vi "Configure Time Interval Gate.vi"(8 "error in (no error)":errorcluster, 9 "Gate Polarity (1: Negative)":i32(ring)=1 items=["Positive", "Negative"], 10 "Gate Source (0: Immediate)":i32(ring) items=["Immediate", "External", "Advanced"], 11 "VISA resource name":refnum<visa-resource-name>) -> (0 "error out":errorcluster, 3 "VISA resource name out":refnum<visa-resource-name>)   [LabVIEW 2021, in "Agilent 532XX Series.lvlib"]
doc: "Configures thecharacteristics of time interval gate.\n\n<B>Note:</B> This VI only applies to the Agilent 53220A/53230A."
uses:
  <instrlib>/Agilent 532XX Series/Agilent 532XX Series.lvlib
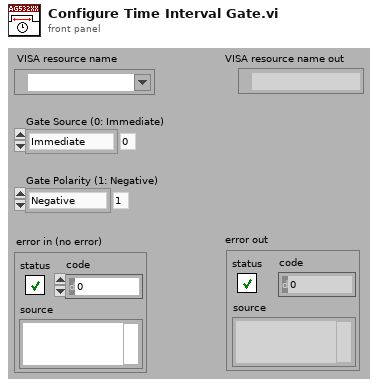
[diagram p1: front panel]
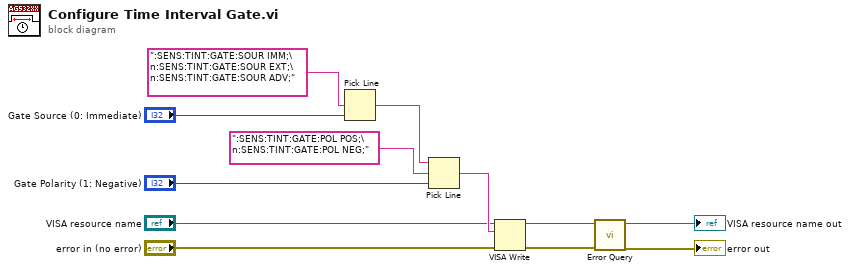
[diagram p0: block diagram]
diagram:
  n1 = Pick Line(multi-line string=":SENS:TINT:GATE:SOUR IMM;\n:SENS:TINT:GATE:SOUR EXT;\n:SENS:TINT:GATE:SOUR ADV;", line index="Gate Source (0: Immediate)") -> (output string=w8:string)  [unwired: 1 out]
  n2 = Pick Line(string ("")=w8, multi-line string=":SENS:TINT:GATE:POL POS;\n:SENS:TINT:GATE:POL NEG;", line index="Gate Polarity (1: Negative)") -> (output string=w7:string)
  n3 = VISA Write(VISA resource name="VISA resource name", write buffer=w7, error in (no error)="error in (no error)") -> (VISA resource name out=w4:refnum<visa-resource-name>, error out=w3:errorcluster)  [unwired: 1 out]
  n4 = call <instrlib>:"Error Query.vi"("error in (no error)"=w3, "VISA resource name"=w4) -> ("error out"=→"error out":errorcluster, "VISA resource name out"=→"VISA resource name out":refnum<visa-resource-name>)  [unwired: 8 out]
